vi "GPIO.vi"(11 "AnalogIn in":refnum<class "AI.lvclass">) -> (2 "GPIO":refnum<class "GPIO.lvclass">)   [LabVIEW 2020, in "CTI.lvlib" / "AI.lvclass"]
uses:
  AI.lvclass
  AI.lvclass/AI.ctl
  GPIO/GPIO.lvclass
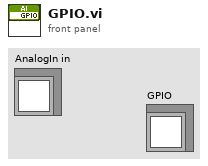
[diagram p1: front panel]
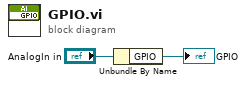
[diagram p0: block diagram]
diagram:
  n1 = Unbundle By Name("AnalogIn in") -> ("GPIO"=→"GPIO":refnum<class "GPIO.lvclass">)
